vi "日報表New20150115.vi"(9 "End Date":string="2014/11/13") -> (0 "error out 2":errorcluster)   [LabVIEW 2012]
uses:
  <vilib>/Utility/NIReport.llb/NI_report.lvclass
  <vilib>/Utility/NIReport.llb/Append Text Table to Report (wrap).vi
  <vilib>/Utility/NIReport.llb/Excel/NI_Excel.lvclass
  <vilib>/addons/_office/NI_ReportGenerationToolkit.lvlib
panel:
  out "error out":errorcluster
  in  "ShiftB":string[][](array[string])
  in  "ShiftA":string[][](array[string])
  in  "ShiftC":string[][](array[string])
  in  "Summary":string[][](array[string])
  out "Row Headers":string[](array[string])
  in  "MonthToDate":string[][](array[string])
  in  "Summary 2":string[][](array[string])
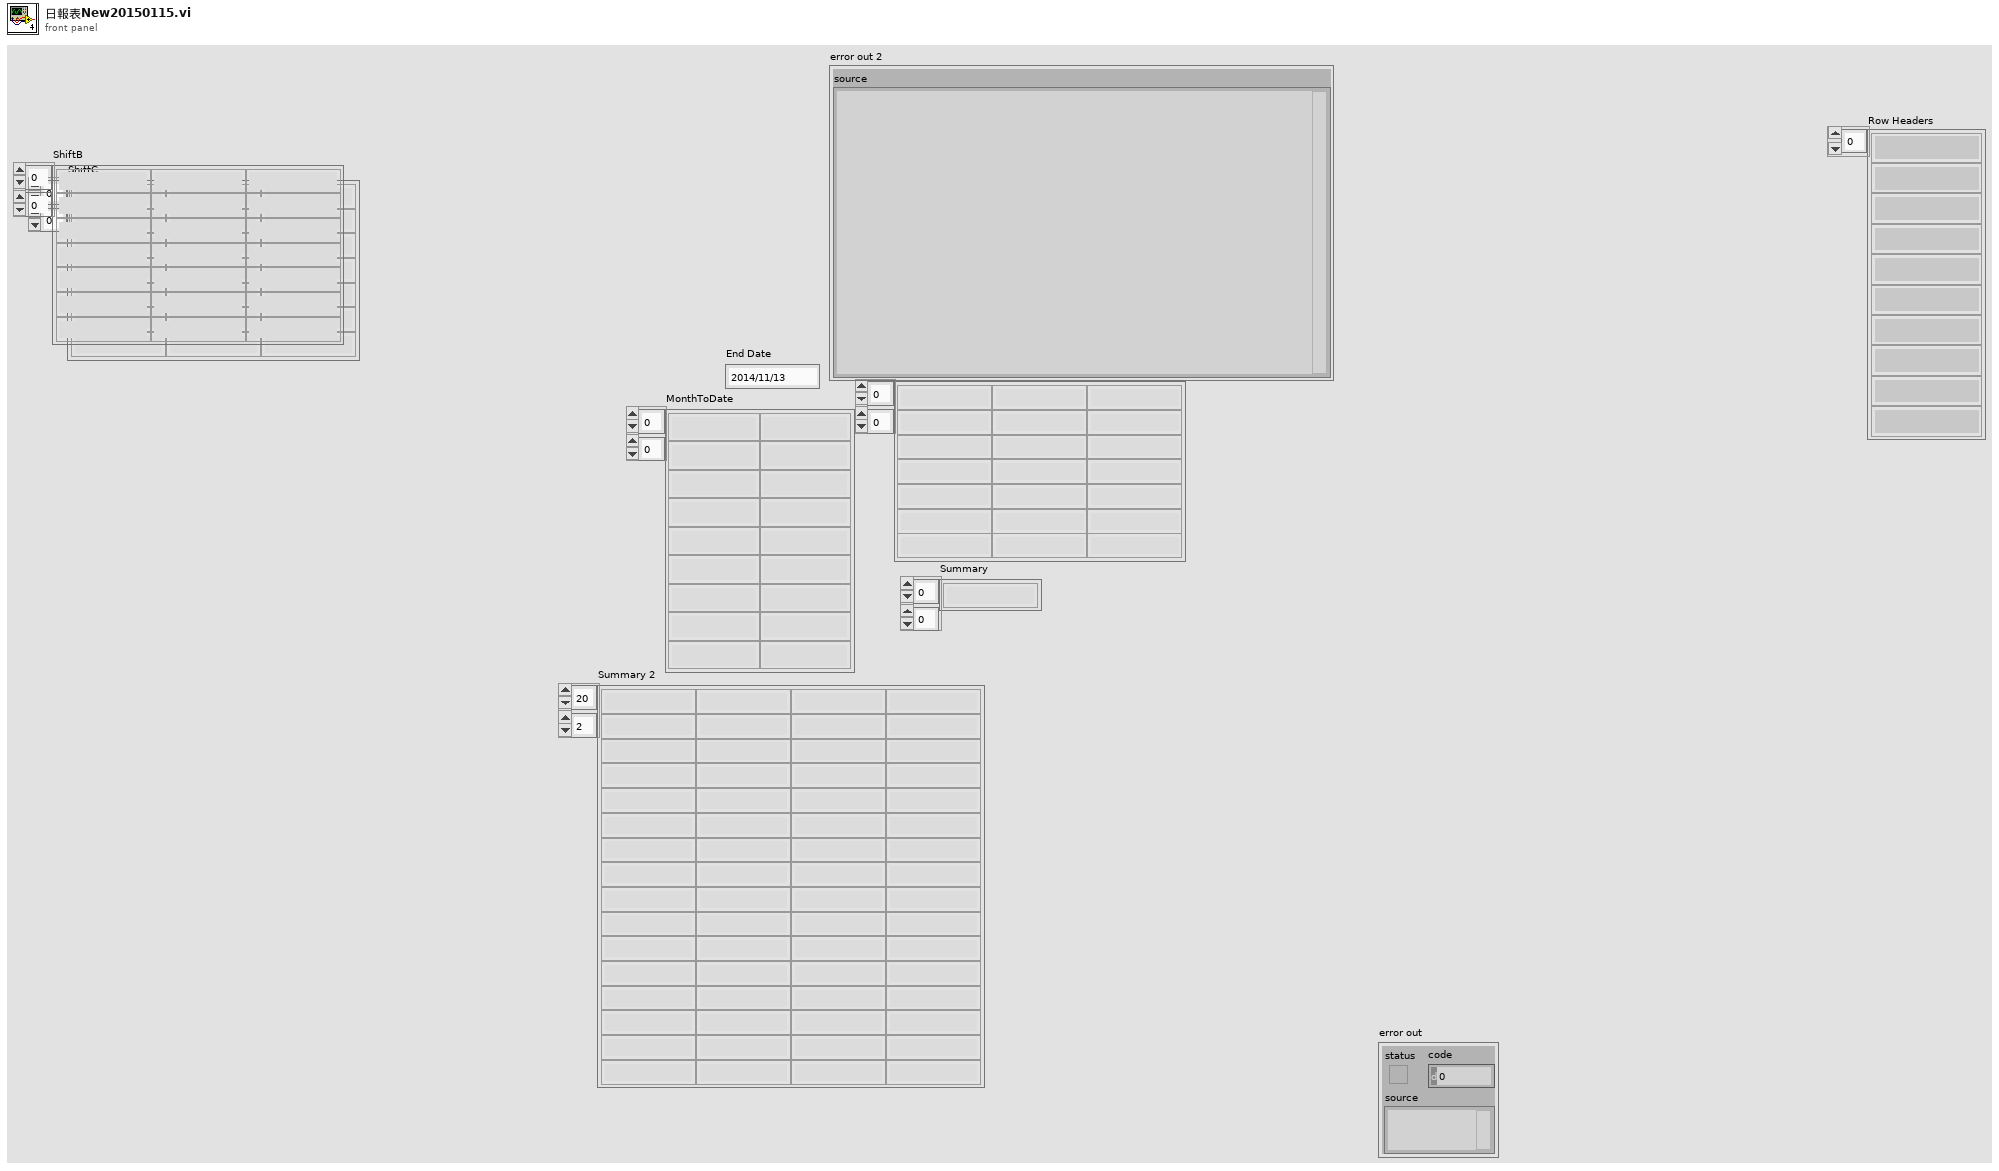
[diagram p1: front panel]
types:
  T1 = enum16{"Standard Report", "HTML", "Word", "Excel"}
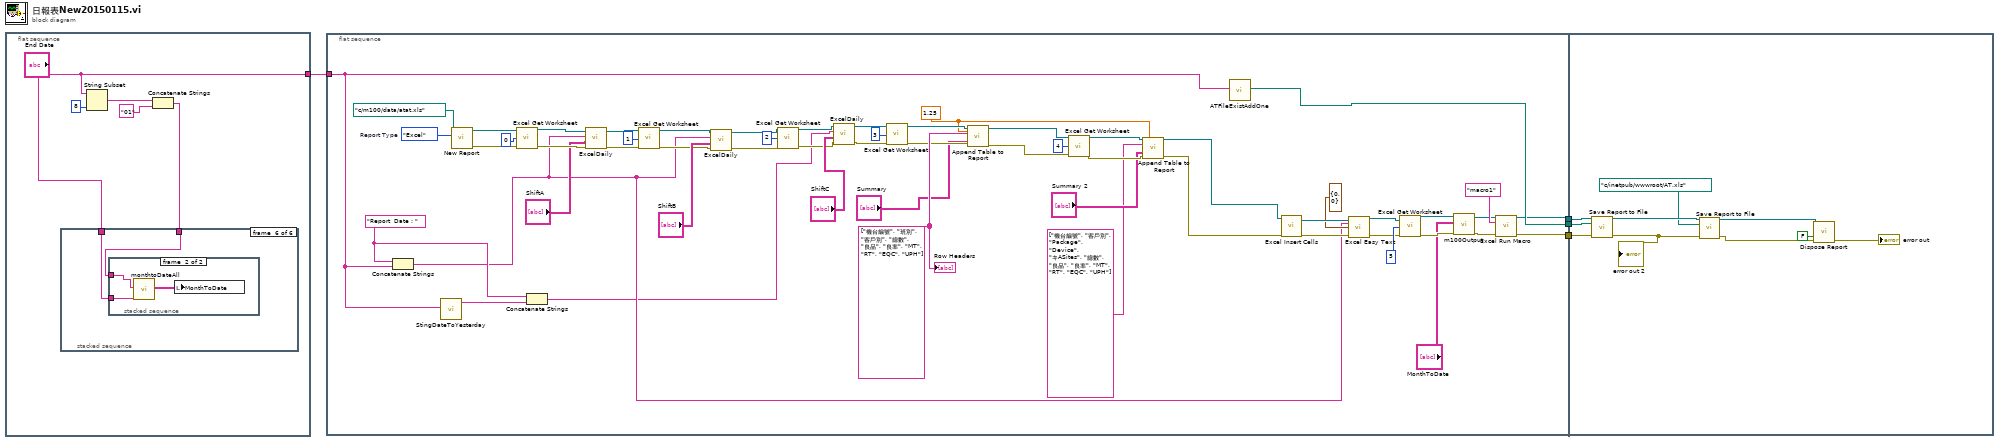
[diagram p0: block diagram]
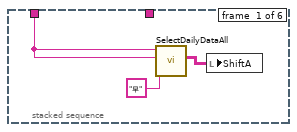
[diagram p2: hidden frame]
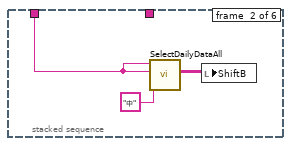
[diagram p3: hidden frame]
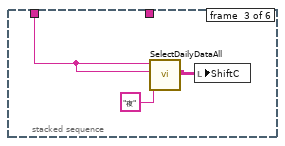
[diagram p4: hidden frame]
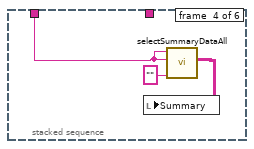
[diagram p5: hidden frame]
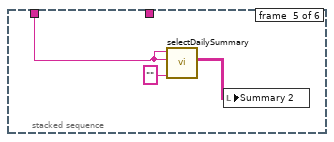
[diagram p6: hidden frame]
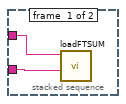
[diagram p7: hidden frame]
diagram:
  n1 = flat-sequence {
    tunnel: ["End Date"] -> w1
    frame #0 {
      n2 = String Subset(string="End Date", length (rest)=8 ("length (rest)")) -> (substring=w8:string)  [unwired: 1 in]
      n3 = Concatenate Strings(w8, "01" ("string")) -> (w6:string)
      n4 = stacked-sequence {
        tunnel: w6 -> [_ _ _ _ _ w25]
        tunnel: "End Date" -> [w10 w13 w16 w19 w23 w26]
        frame #0 {
          n5 = call "SelectDailyDataAll.vi"("Shift"="早", "End_date"=w10, "Begin_date"=w10) -> ("output array"=w11:string[][])  [unwired: 8 in]
          n6 = local write "ShiftA"(w11) -> ()
        }
        frame #1 {
          n7 = call "SelectDailyDataAll.vi"("Shift"="中", "End_date"=w13, "Begin_date"=w13) -> ("output array"=w14:string[][])  [unwired: 8 in]
          n8 = local write "ShiftB"(w14) -> ()
        }
        frame #2 {
          n9 = call "SelectDailyDataAll.vi"("Shift"="夜", "End_date"=w16, "Begin_date"=w16) -> ("output array"=w17:string[][])  [unwired: 8 in]
          n10 = local write "ShiftC"(w17) -> ()
        }
        frame #3 {
          n11 = call "selectSummaryDataAll.vi"("Shift"="", "End_date"=w19, "Begin_date"=w19) -> ("Summary"=w21:string[][])  [unwired: 8 in]
          n12 = local write "Summary"(w21) -> ()
        }
        frame #4 {
          n13 = call "selectDailySummary.vi"("Shift"="", "End_date"=w23, "Begin_date"=w23) -> ("Summary"=w22:string[][])  [unwired: 8 in]
          n14 = local write "Summary 2"(w22) -> ()
        }
        frame #5 {
          n15 = stacked-sequence {
            tunnel: w26 -> [w28 w29]
            tunnel: w25 -> [w27 w30]
            frame #0 {
              n16 = call "loadFTSUM.vi"("End Date"=w28, "From Date"=w27) -> ()  [unwired: 9 in, 1 out]
            }
            frame #1 {
              n17 = call "monthtoDateAll.vi"("End Date"=w29, "From Date"=w30) -> ("output array"=w31:string[][])  [unwired: 8 in, 1 out]
              n18 = local write "MonthToDate"(w31) -> ()
            }
          }
        }
      }
    }
  }
  n19 = flat-sequence {
    tunnel: w1 -> [w54]
    tunnel: [w33] -> w4
    tunnel: [w32] -> w3
    tunnel: [w55] -> w2
    tunnel: w4 -> [w98]
    tunnel: w3 -> [w97]
    tunnel: w2 -> [w96]
    frame #0 {
      w52 = "Report  Date : " ("string")
      w66 = string[] ["機台編號", "班別", "客戶別", "總數", "良品", "良率", "MT", "RT", "EQC", "UPH"] ("row headers")
      w43 = 1.25 ("column width (1)")
      w88 = T1."Excel"  # Report Type
      n20 = Concatenate Strings(w52, w54) -> (w51:string)
      n21 = call "StingDateToYesterday.vi"("Date"=w54) -> ("Date+1"=w53:string)  [unwired: 9 in, 1 out]
      n22 = call <vilib>:"New Report.vi"("report type"=w88, "template (empty)"=path "c:/m100/data/atat.xls") -> ("report out"=w87:refnum<class "NI_report.lvclass">, "error out"=w86:errorcluster)  [unwired: 12 in]
      n23 = call <vilib>:"Excel Get Worksheet.vi"("report in"=w87, "worksheet index (0)"=0, "error in (no error)"=w86) -> ("report out"=w84:refnum<class "NI_report.lvclass">, "error out"=w83:errorcluster)  [unwired: 11 in]
      n24 = Concatenate Strings(w52, w53) -> (w50:string)
      n25 = call "ExcelDaily.vi"("error in (no error)"=w83, "Input"="ShiftA", "Header"=w51, "report in"=w84) -> ("error out"=w77:errorcluster, "report out"=w79:refnum<class "NI_report.lvclass">)  [unwired: 6 in]
      n26 = call <vilib>:"Excel Get Worksheet.vi"("report in"=w79, "worksheet index (0)"=1, "error in (no error)"=w77) -> ("report out"=w78:refnum<class "NI_report.lvclass">, "error out"=w76:errorcluster)  [unwired: 11 in]
      n27 = call "ExcelDaily.vi"("error in (no error)"=w76, "Input"="ShiftB", "Header"=w51, "report in"=w78) -> ("error out"=w73:errorcluster, "report out"=w74:refnum<class "NI_report.lvclass">)  [unwired: 6 in]
      n28 = call <vilib>:"Excel Get Worksheet.vi"("report in"=w74, "worksheet index (0)"=2, "error in (no error)"=w73) -> ("report out"=w72:refnum<class "NI_report.lvclass">, "error out"=w71:errorcluster)  [unwired: 11 in]
      n29 = call "ExcelDaily.vi"("error in (no error)"=w71, "Input"="ShiftC", "Header"=w50, "report in"=w72) -> ("error out"=w68:errorcluster, "report out"=w69:refnum<class "NI_report.lvclass">)  [unwired: 6 in]
      n30 = call <vilib>:"Excel Get Worksheet.vi"("report in"=w69, "worksheet index (0)"=3, "error in (no error)"=w68) -> ("report out"=w62:refnum<class "NI_report.lvclass">, "error out"=w61:errorcluster)  [unwired: 11 in]
      n31 = call-poly <vilib>:"Append Table to Report.vi"("report in"=w62, "column width (1)"=w43, "column headers"=w66, "text data"="Summary", "error in (no error)"=w61) -> ("report out"=w49:refnum<class "NI_report.lvclass">, "error out"=w48:errorcluster)  [unwired: 7 in, 2 out]
      n32 = call <vilib>:"Excel Get Worksheet.vi"("report in"=w49, "worksheet index (0)"=4, "error in (no error)"=w48) -> ("report out"=w46:refnum<class "NI_report.lvclass">, "error out"=w45:errorcluster)  [unwired: 11 in]
      n33 = call-poly <vilib>:"Append Table to Report.vi"("report in"=w46, "column width (1)"=w43, "column headers"=string[] ["機台編號", "客戶別", "Package", "Device", "キАSites", "總數", "良品", "良率", "MT", "RT", "EQC", "UPH"] ("row headers"), "text data"="Summary 2", "error in (no error)"=w45) -> ("report out"=w42:refnum<class "NI_report.lvclass">, "error out"=w41:errorcluster)  [unwired: 7 in, 2 out]
      n34 = call "ATFileExistAddOne.vi"("input string"=w54) -> ("appended path"=w55:path)  [unwired: 10 in]
      n35 = call <vilib>:"Excel Insert Cells.vi"("report in"=w42, "error in (no error)"=w41) -> ("report out"=w65:refnum<class "NI_report.lvclass">, "error out"=w64:errorcluster)  [unwired: 12 in]
      n36 = call <vilib>:"Excel Easy Text.vi"("report in"=w65, "text"=w51, "start (-1, -1)"=cluster{"row":i32, "column":i32} {"row"=0, "column"=0} ("end (-1, -1)"), "error in (no error)"=w64) -> ("report out"=w38:refnum<class "NI_report.lvclass">, "error out"=w37:errorcluster)  [unwired: 7 in, 3 out]
      n37 = call <vilib>:"Excel Get Worksheet.vi"("report in"=w38, "worksheet index (0)"=5, "error in (no error)"=w37) -> ("report out"=w58:refnum<class "NI_report.lvclass">, "error out"=w57:errorcluster)  [unwired: 11 in]
      n38 = call "m100Output.vi"("error in (no error)"=w57, "Input"="MonthToDate", "report in"=w58) -> ("error out"=w34:errorcluster, "report out"=w35:refnum<class "NI_report.lvclass">)  [unwired: 7 in]
      n39 = call <vilib>:"Excel Run Macro.vi"("report in"=w35, "macro name"="macro1", "error in (no error)"=w34) -> ("report out"=w33:refnum<class "NI_report.lvclass">, "error out"=w32:errorcluster)  [unwired: 10 in, 1 out]
      "Row Headers" <- w66
    }
    frame #1 {
      n40 = call-dynamic "Save Report to File.vi"("report in"=w98, "report file path"=w96, "error in (no error)"=w97) -> ("report out"=w93:refnum<class "NI_report.lvclass">, "error out"=w91:errorcluster)  [unwired: 11 in]
      "error out 2" <- w91
      n41 = call-dynamic "Save Report to File.vi"("report in"=w93, "report file path"=path "c:/inetpub/wwwroot/AT.xls", "error in (no error)"=w91) -> ("report out"=w92:refnum<class "NI_report.lvclass">, "error out"=w90:errorcluster)  [unwired: 11 in]
      n42 = call-dynamic "Dispose Report.vi"("report in"=w92, "save changes? (F)"=FALSE, "error in (no error)"=w90) -> ("error out"=→"error out":errorcluster)  [unwired: 12 in]
    }
  }
